vi "8_Flicker.vi"(9 "Remote IP Address":string="10.1.21.134") -> (0 "error out":errorcluster, 3 "FLICKER Tüm Fazlar":sgl[][](array[numeric]) format="%_5g")   [LabVIEW 2014]
panel:
  out "Flicker FD2 Vc":sgl format="%_5f"
  out "Flicker FD2 Vb":sgl format="%_5f"
  out "Flicker FD2 Va":sgl format="%_5f"
  out "Flicker FD1 Vc":sgl format="%_5f"
  out "Flicker FD1 Vb":sgl format="%_5f"
  out "Flicker FD1 Va":sgl format="%_5f"
  in  "Flicker FD2 Vc Register":u16=683
  in  "Flicker FD2 Vb Register":u16=681
  in  "Flicker FD2 Va Register":u16=679
  in  "Flicker FD1 Vc Register":u16=19
  in  "Flicker FD1 Vb Register":u16=17
  in  "Flicker FD1 Va Register":u16=15
  out "time stamp":timestamp=timestamp(1426515300 s since 1904-01-01) format="%<%H:%M:%S>T"
  in  "Remote Port":u16=1502
  # "MB Ethernet Example Master.vi\n\nInstructions\n1. Run MB Ethernet Example Slave.vi\n2. Run this VI.\n3. Modify the discrete inputs or input registers on the slave -> they're updated on the master.\n4. Modify the coils and registers on the master -> they're updated on the slave."
  # "TCP Parameters"
  # "Slave Read-only Registers"
  # "FD1 Psta"
  # "FD1 Pstb"
  # "FD1 Pstc"
  # "FD2 Psta"
  # "FD2 Pstb"
  # "FD2 Pstc"
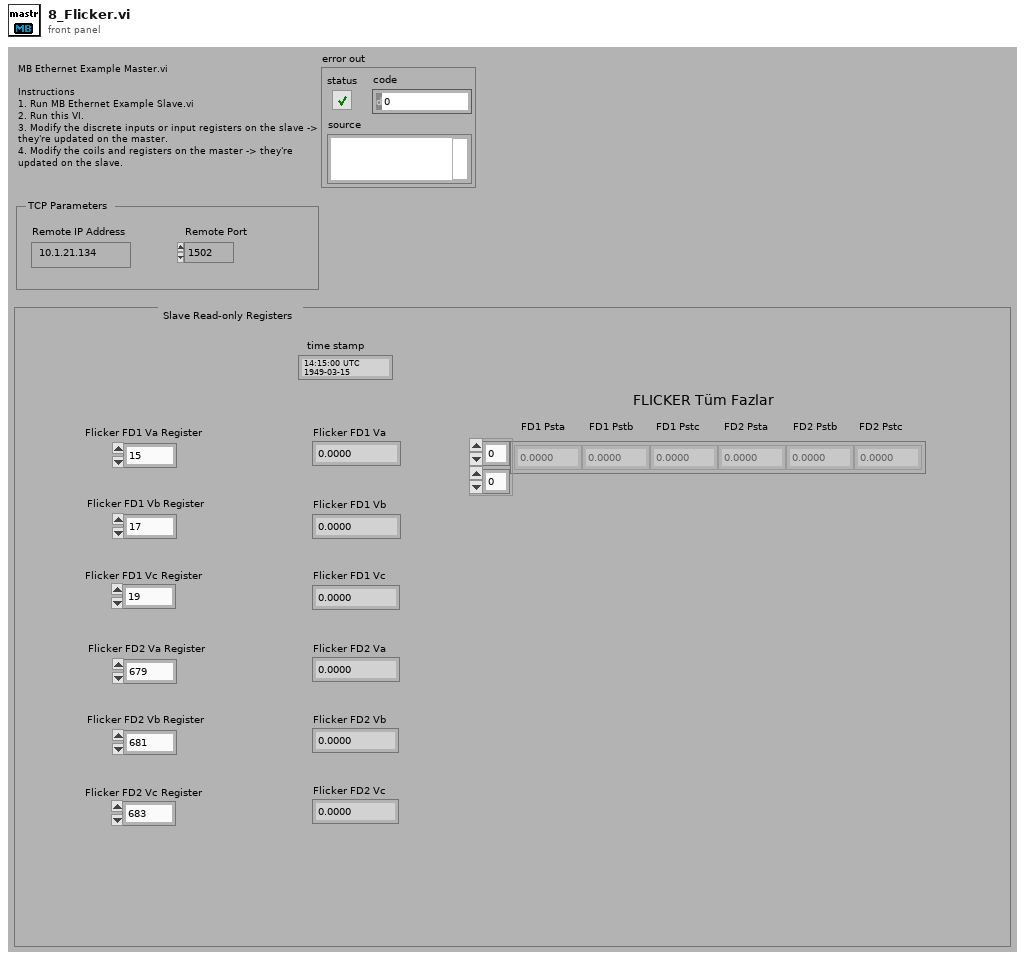
[diagram p1: front panel]
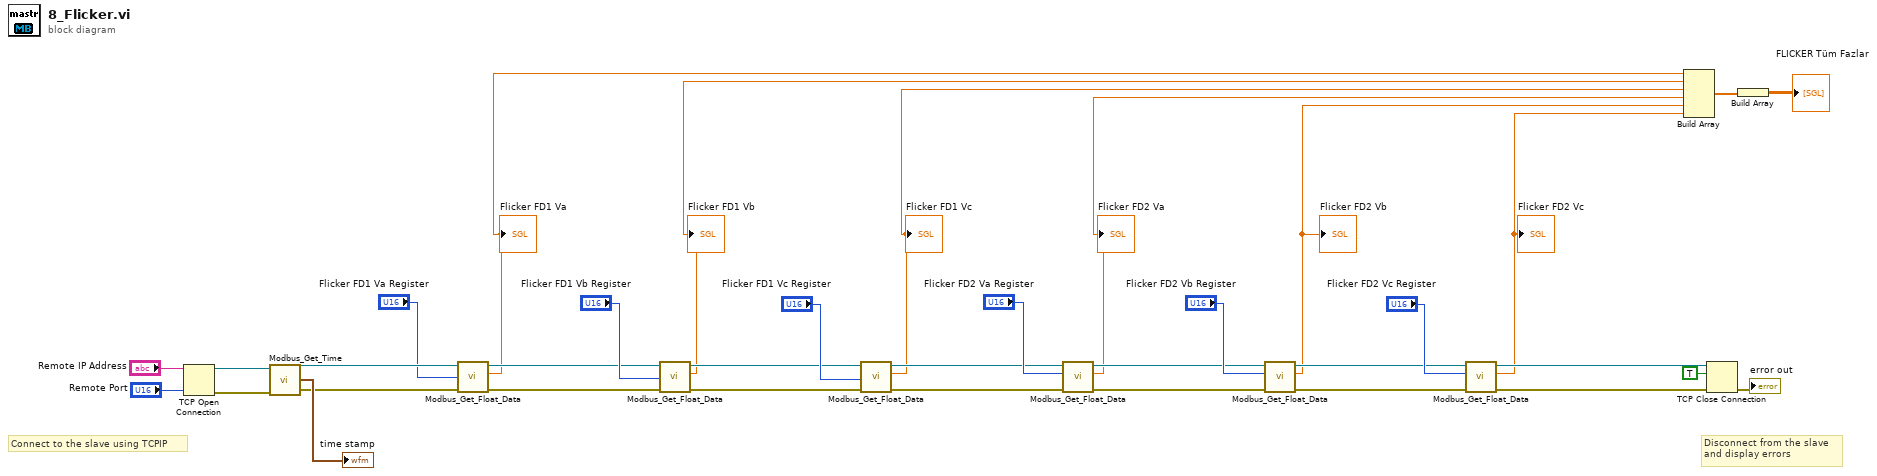
[diagram p0: block diagram]
diagram:
  # "Disconnect from the slave\nand display errors"
  # "Connect to the slave using TCPIP"
  n1 = TCP Open Connection(address="Remote IP Address", remote port or service name="Remote Port") -> (connection ID=w33:refnum<k5>, error out=w32:errorcluster)  [unwired: 1 in, 2 out]
  n2 = call "Modbus_Get_Time.vi"("error in (no error)"=w32, "TCP Network Connection in"=w33) -> ("error out"=w24:errorcluster, "Time Stamp"=→"time stamp":timestamp, "TCP Network Connection out"=w26:refnum<k5>)  [unwired: 6 in, 1 out]
  n3 = call "Modbus_Get_Float_Data.vi"("error in (no error)"=w24, "Starting Address (2 Bytes)"="Flicker FD1 Va Register", "TCP Network Connection in"=w26) -> ("error out"=w22:errorcluster, "Numeric"=w8:sgl, "TCP Network Connection out"=w21:refnum<k5>)  [unwired: 5 in, 1 out]
  "Flicker FD1 Va" <- w8
  n4 = call "Modbus_Get_Float_Data.vi"("error in (no error)"=w22, "Starting Address (2 Bytes)"="Flicker FD1 Vb Register", "TCP Network Connection in"=w21) -> ("error out"=w19:errorcluster, "Numeric"=w7:sgl, "TCP Network Connection out"=w18:refnum<k5>)  [unwired: 5 in, 1 out]
  "Flicker FD1 Vb" <- w7
  n5 = call "Modbus_Get_Float_Data.vi"("error in (no error)"=w19, "Starting Address (2 Bytes)"="Flicker FD1 Vc Register", "TCP Network Connection in"=w18) -> ("error out"=w14:errorcluster, "Numeric"=w6:sgl, "TCP Network Connection out"=w11:refnum<k5>)  [unwired: 5 in, 1 out]
  "Flicker FD1 Vc" <- w6
  n6 = call "Modbus_Get_Float_Data.vi"("error in (no error)"=w14, "Starting Address (2 Bytes)"="Flicker FD2 Va Register", "TCP Network Connection in"=w11) -> ("error out"=w13:errorcluster, "Numeric"=w5:sgl, "TCP Network Connection out"=w10:refnum<k5>)  [unwired: 5 in, 1 out]
  "Flicker FD2 Va" <- w5
  n7 = call "Modbus_Get_Float_Data.vi"("error in (no error)"=w13, "Starting Address (2 Bytes)"="Flicker FD2 Vb Register", "TCP Network Connection in"=w10) -> ("error out"=w12:errorcluster, "Numeric"=w4:sgl, "TCP Network Connection out"=w9:refnum<k5>)  [unwired: 5 in, 1 out]
  "Flicker FD2 Vb" <- w4
  n8 = call "Modbus_Get_Float_Data.vi"("error in (no error)"=w12, "Starting Address (2 Bytes)"="Flicker FD2 Vc Register", "TCP Network Connection in"=w9) -> ("error out"=w31:errorcluster, "Numeric"=w3:sgl, "TCP Network Connection out"=w28:refnum<k5>)  [unwired: 5 in, 1 out]
  "Flicker FD2 Vc" <- w3
  n9 = Build Array(w8, w7, w6, w5, w4, w3) -> (w2:sgl[])
  n10 = TCP Close Connection(connection ID=w28, abort (F)=TRUE, error in (no error)=w31) -> (error out=→"error out":errorcluster)  [unwired: 1 out]
  n11 = Build Array(w2) -> (→"FLICKER Tüm Fazlar":sgl[][])
